vi "TCP Transmit Message.vi"(7 "Magic":u32=3737844653 format="%x", 8 "Error In":errorcluster, 9 "Wait for response":bool, 10 "Message":string, 11 "connection ID":refnum<k5>) -> (0 "Error Out":errorcluster, 1 "Valid response":bool, 2 "Response":string, 3 "connection ID out":refnum<k5>)   [LabVIEW 2019]
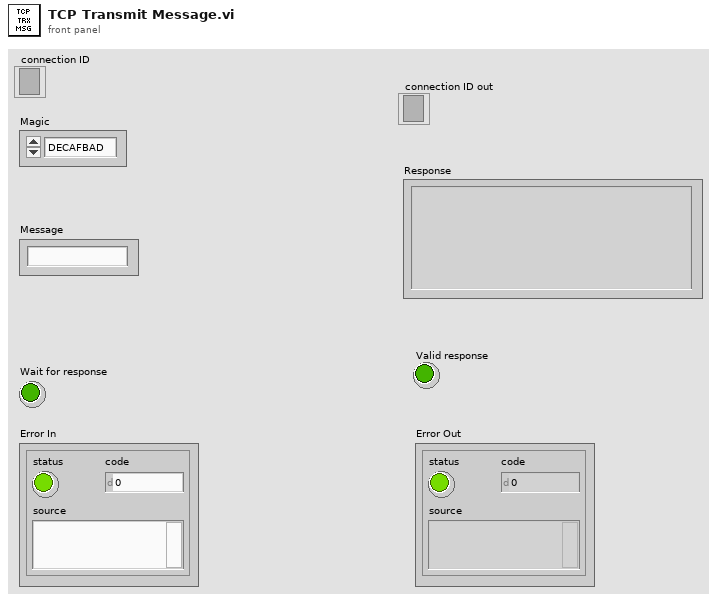
[diagram p1: front panel]
types:
  T1 = enum16{"big-endian, network order", "native, host order", "little-endian"}
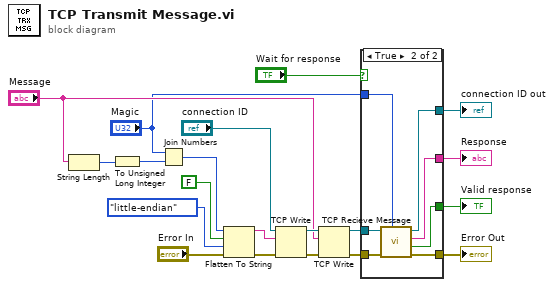
[diagram p0: block diagram]
diagram:
  n1 = String Length(string="Message") -> (length=w20:i32)
  n2 = To Unsigned Long Integer(number=w20) -> (unsigned 32bit integer=w19:u32)
  n3 = Join Numbers(hi="Magic", lo=w19) -> ((hi.lo)=w17:u64)
  n4 = Flatten To String(anything=w17, prepend array or string size? (T)=FALSE, byte order (0:big-endian, network order)=T1."little-endian", error in (no error)="Error In") -> (data string=w13:string, error out=w16:errorcluster)  [unwired: 1 out]
  n5 = TCP Write(connection ID="connection ID", data in=w13, error in (no error)=w16) -> (connection ID out=w11:refnum<k5>, error out=w12:errorcluster)  [unwired: 1 in, 1 out]
  n6 = TCP Write(connection ID=w11, data in="Message", error in (no error)=w12) -> (connection ID out=w6:refnum<k5>, error out=w7:errorcluster)  [unwired: 1 in, 1 out]
  n7 = case shown="True" "Wait for response" {
    tunnel: w7 -> [w22 w27]
    tunnel: w6 -> [w21 w29]
    tunnel: [w21 w28] -> w5
    tunnel: [w22 w26] -> w4
    tunnel: [_ w25] -> w3
    tunnel: [_ w24] -> w2
    tunnel: "Magic" -> [_ w23]
    frame False {
    }
    frame True {
      n8 = call "TCP Recieve Message.vi"("Magic"=w23, "Error In"=w27, "connection ID"=w29) -> ("Error Out"=w26:errorcluster, "Valid"=w25:bool, "Response"=w24:string, "connection ID out"=w28:refnum<k5>)  [unwired: 5 in]
    }
  }
  "Error Out" <- w4
  "connection ID out" <- w5
  "Valid response" <- w3
  "Response" <- w2
